vi "Maximize.vi"(8 "error in":errorcluster, 11 "Philips UI in":refnum<class "Flex UI.lvclass">) -> (0 "error out":errorcluster, 3 "Philips UI out":refnum<class "Flex UI.lvclass">)   [LabVIEW 2014, in "Flex UI.lvclass"]
doc: "Maximizes the UI."
uses:
  Flex UI.lvclass
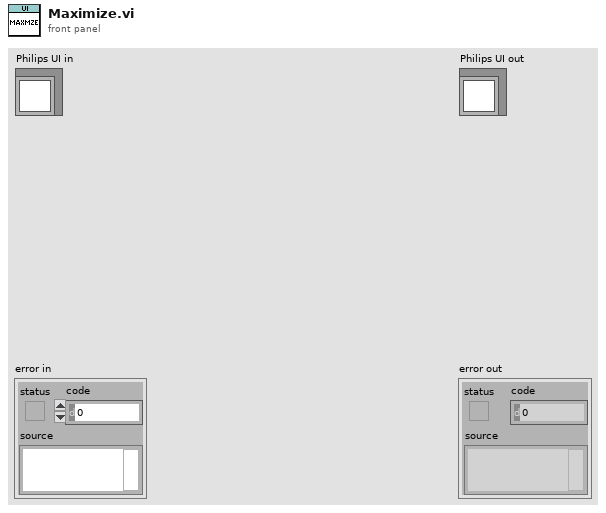
[diagram p1: front panel]
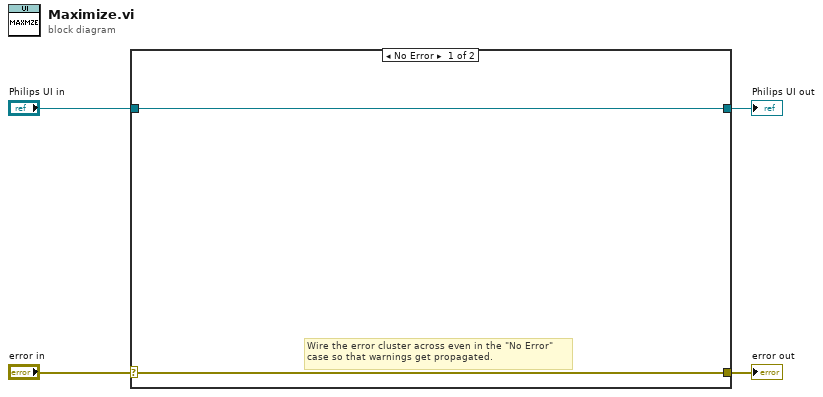
[diagram p0: block diagram]
diagram:
  n1 = case shown="No Error" "error in" {
    selector: "error in" -> [w5 w8]
    tunnel: [w5 w8] -> w3
    tunnel: [w6 w7] -> w1
    tunnel: "Philips UI in" -> [w6 w7]
    frame No Error {
      # "Wire the error cluster across even in the \"No Error\"\ncase so that warnings get propagated."
    }
    frame Error {
    }
  }
  "error out" <- w3
  "Philips UI out" <- w1
